vi "applyDM_and_acqTIFF.vi"(0 "EMCCD trigger port":tag="Dev1/port0/line0", 1 "WavefrontCorrector in":refnum<class "WavefrontCorrector.lvclass">, 3 "Absolute Positions":T1, 5 "exp and readout time (ms)":dbl, 9 "Img Num":i32, 11 "error in (no error)":errorcluster, 12 "strPath":string="_groundtruth_", 13 "Clean Spooling":bool=TRUE, 14 "strPalette":string="_groundtruth_") -> (4 "WavefrontCorrector out":refnum<class "WavefrontCorrector.lvclass">, 15 "error out":errorcluster)   [LabVIEW 2018]
uses:
  <userlib>/WaveKit.lib/Classes/WavefrontCorrector/WavefrontCorrector.lvclass
  <userlib>/WaveKit.lib/Controls/Wavefront Corrector Position.ctl
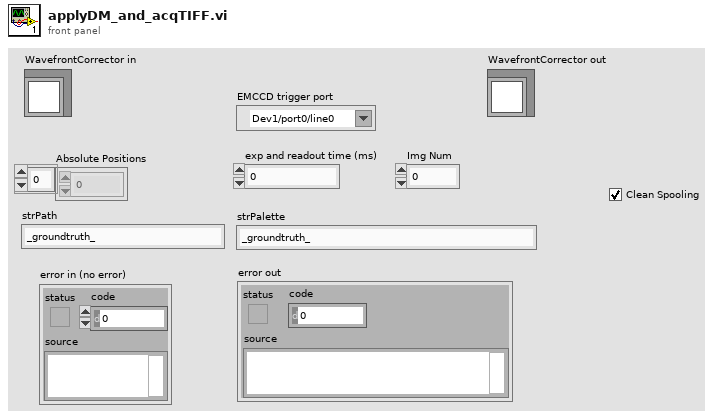
[diagram p1: front panel]
types:
  T1 = typedef "Wavefront Corrector Position.ctl" = sgl[]
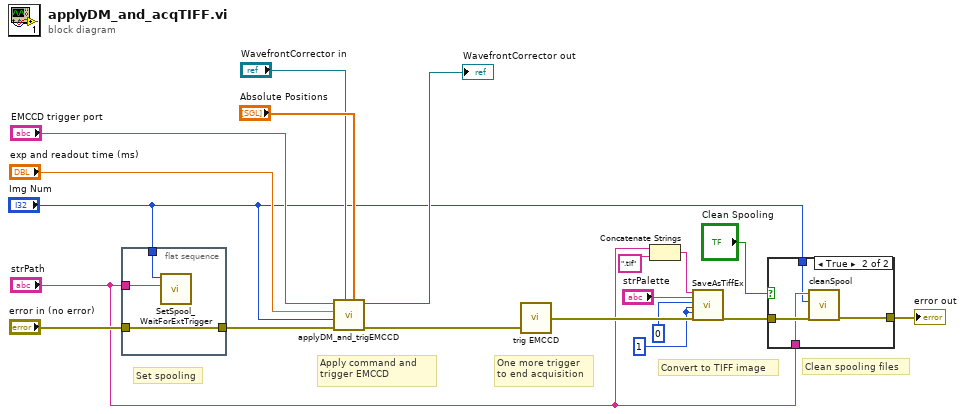
[diagram p0: block diagram]
diagram:
  w12 = 1
  # "Apply command and \ntrigger EMCCD"
  # "Set spooling"
  # "Clean spooling files"
  # "Convert to TIFF image"
  # "One more trigger\nto end acquisition"
  n1 = flat-sequence {
    tunnel: "strPath" -> [w22]
    tunnel: "Img Num" -> [w21]
    tunnel: "error in (no error)" -> [w20]
    tunnel: [w20] -> w9
    frame #0 {
      n2 = call "SetSpool_WaitForExtTrigger.vi"("path and name"=w22, "Kinetic Series"=w21) -> ()  [unwired: 10 in]
    }
  }
  n3 = call "applyDM_and_trigEMCCD.vi"("Absolute Positions"="Absolute Positions", "WavefrontCorrector in"="WavefrontCorrector in", "error in (no error)"=w9, "Trig Num"="Img Num", "exp and readout time (ms)"="exp and readout time (ms)", "EMCCD trigger port"="EMCCD trigger port") -> ("error out"=w7:errorcluster, "WavefrontCorrector out"=→"WavefrontCorrector out":refnum<class "WavefrontCorrector.lvclass">)  [unwired: 4 in]
  n4 = call "trig EMCCD.vi"("error in (no error)"=w7) -> ("error out"=w15:errorcluster)  [unwired: 2 in]
  n5 = Concatenate Strings("strPath", ".tif") -> (w14:string)
  n6 = call <userlib>:"SaveAsTiffEx.vi"("path"=w14, "palette"="strPalette", "position"=0, "type"=w12, "mode"=w12, "error in (no error)"=w15) -> ("error out"=w5:errorcluster)  [unwired: 12 in, 1 out]
  n7 = case shown="True" "Clean Spooling" {
    tunnel: w5 -> [w23 w27]
    tunnel: [w23 w26] -> w4
    tunnel: "strPath" -> [_ w25]
    tunnel: "Img Num" -> [_ w24]
    frame False {
    }
    frame True {
      n8 = call "cleanSpool.vi"("error in (no error)"=w27, "Total Img Num"=w24, "strPath"=w25) -> ("error out"=w26:errorcluster)  [unwired: 8 in]
    }
  }
  "error out" <- w4
